vi "ts_tree_set_msg.vi"(8 "error in (no error)":errorcluster, 10 "msg":string, 11 "Tree.in":refnum<vi>) -> (0 "error out":errorcluster, 3 "Tree.out":refnum<vi>)   [LabVIEW 2015]
doc: "sets the test step description in the tree control, ignares comments (#) and child test steps($)"
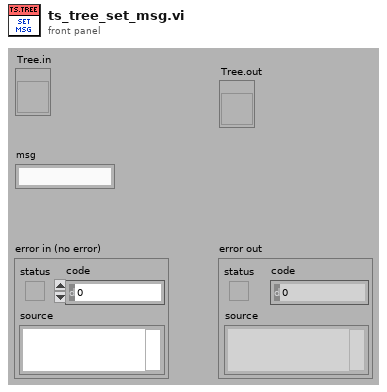
[diagram p1: front panel]
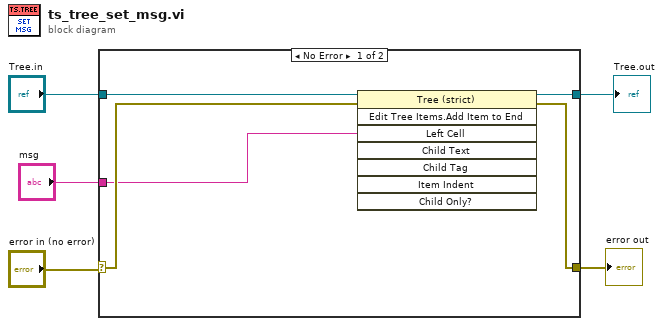
[diagram p0: block diagram]
diagram:
  n1 = case shown="No Error" "error in (no error)" {
    selector: "error in (no error)" -> [w8 w11]
    tunnel: "Tree.in" -> [w10 w12]
    tunnel: [w9 w12] -> w3
    tunnel: [w7 w11] -> w2
    tunnel: "msg" -> [w6 _]
    frame No Error {
      n2 = invoke class="Tree (strict)" method="Edit Tree Items.Add Item to End"(reference=w10, error in=w8, "Left Cell"=w6) -> (reference out=w9:refnum<vi>, error out=w7:errorcluster)  [unwired: 5 in, 6 out]
    }
    frame Error {
    }
  }
  "Tree.out" <- w3
  "error out" <- w2
